vi "Agilent 3631A Initialize.vi"(8 "error in (no error)":errorcluster, 9 "Default":bool, 10 "Reset":bool, 11 "VISA resource name":refnum<visa-resource-name>) -> (0 "error out":errorcluster, 3 "VISA resource name out":refnum<visa-resource-name>)   [LabVIEW 2017]
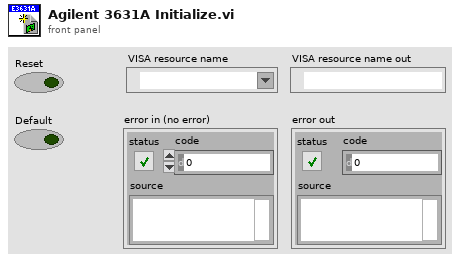
[diagram p1: front panel]
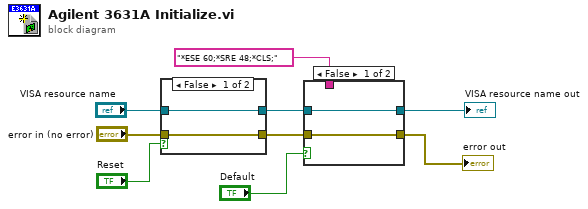
[diagram p0: block diagram]
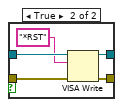
[diagram p2: hidden frame]
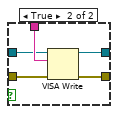
[diagram p3: hidden frame]
diagram:
  n1 = case shown="False" "Reset" {
    tunnel: "VISA resource name" -> [w10 w16]
    tunnel: [w11 w14] -> w7
    tunnel: [w10 w13] -> w6
    tunnel: "error in (no error)" -> [w11 w12]
    frame False {
    }
    frame True {
      n2 = VISA Write(VISA resource name=w16, write buffer="*RST", error in (no error)=w12) -> (VISA resource name out=w13:refnum<visa-resource-name>, error out=w14:errorcluster)  [unwired: 1 out]
    }
  }
  n3 = case shown="False" "Default" {
    tunnel: "*ESE 60;*SRE 48;*CLS;" ("write buffer") -> [_ w23]
    tunnel: w7 -> [w18 w22]
    tunnel: w6 -> [w17 w21]
    tunnel: [w18 w20] -> w4
    tunnel: [w17 w19] -> w3
    frame False {
    }
    frame True {
      n4 = VISA Write(VISA resource name=w21, write buffer=w23, error in (no error)=w22) -> (VISA resource name out=w19:refnum<visa-resource-name>, error out=w20:errorcluster)  [unwired: 1 out]
    }
  }
  "error out" <- w4
  "VISA resource name out" <- w3
